vi "Pockels-Mov cor tracing in funct acq.vi"(6 "Cluster":T1={"Pockels ON \"Pre\" (samples)"=2, "Direction (+-Inf)"=enum."No rounding", "Additional duration to stay ON (samples)"=0, "Not the last ROI"=FALSE}, 7 "Actual component time (us)":dbl, 8 "Count towards trigger target (ms) in":dbl, 10 "Excess (us) in":dbl, 11 "Single ROI pockels modulation AO sequence (in)":dbl[](array[numeric])) -> (0 "Count towards trigger target (ms)":dbl, 2 "Excess (us)":dbl, 3 "AO pockels modulation sequence (out)":dbl[](array[numeric]))   [LabVIEW 2020]
uses:
  Typedefs/Pockels modulation Internal cluster 1.ctl
  Typedefs/Rounding type.ctl
  Typedefs/Imaging Protocols enum.ctl
  Globals/gl_Pockels control globals.vi
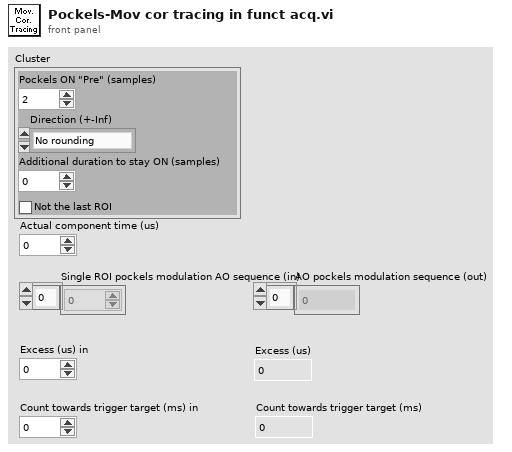
[diagram p1: front panel]
types:
  T1 = typedef "Pockels modulation Internal cluster 1.ctl" = cluster{"Pockels ON \"Pre\" (samples)":i32, "Direction (+-Inf)":T2, "Additional duration to stay ON (samples)":i32, "Not the last ROI":bool}
  T2 = typedef "Rounding type.ctl" = enum16{"No rounding", "Toward +Inf", "Toward -Inf"}
  T3 = typedef "Imaging Protocols enum.ctl" = enum16{"AOL Z-Stack", "Motor Z Stack", "Functional Acquisition", "Single Plane Acquisition", "Volume Acquisition", "Live Imaging", "Live Plane Imaging", "Live Volume Imaging"}
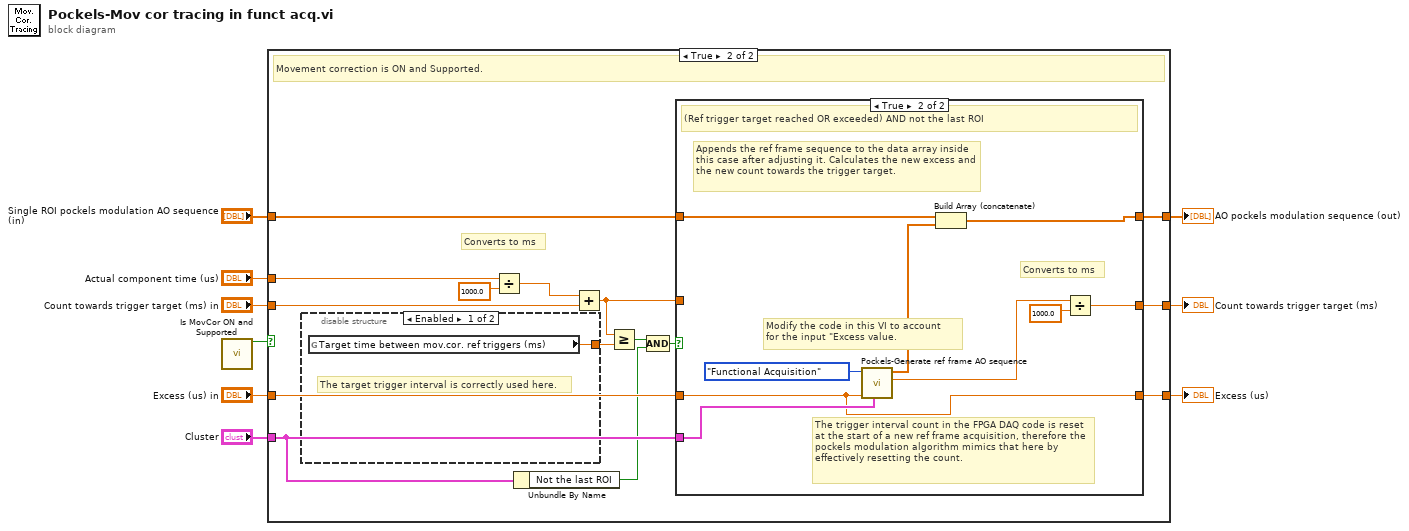
[diagram p0: block diagram]
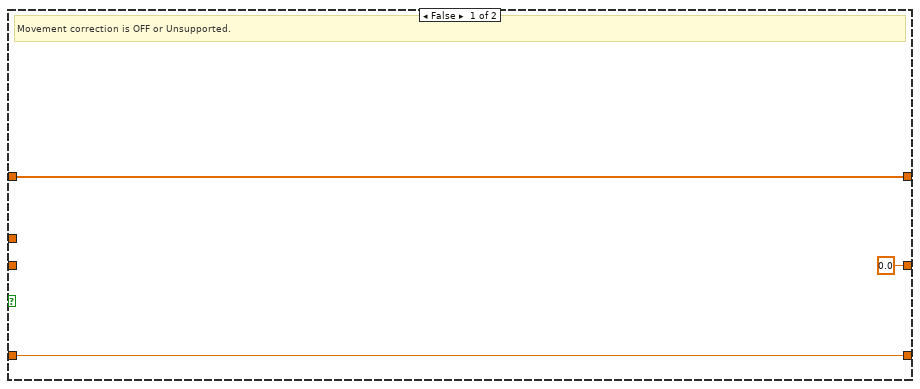
[diagram p2: hidden frame]
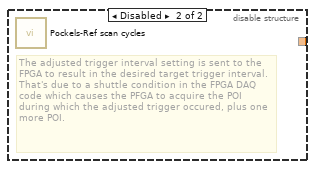
[diagram p3: hidden frame]
diagram:
  n1 = call "Is MovCor ON and Supported.vi"() -> ("MovCor is ON and Supported"=w1:bool)  [unwired: 11 in]
  n2 = case shown="True" w1 {
    tunnel: "Actual component time (us)" -> [_ w26]
    tunnel: "Count towards trigger target (ms) in" -> [_ w24]
    tunnel: "Excess (us) in" -> [w11 w23]
    tunnel: [w11 w22] -> w6
    tunnel: [0.0 w21] -> w5
    tunnel: "Single ROI pockels modulation AO sequence (in)" -> [w12 w20]
    tunnel: [w12 w19] -> w3
    tunnel: "Cluster" -> [_ w14]
    frame False {
      # "Movement correction is OFF or Unsupported."
    }
    frame True {
      # "Converts to ms"
      # "Movement correction is ON and Supported."
      n3 = disable-structure shown="Enabled" {
        disable-tunnel: [w28 _] -> w27
        frame Enabled {
          # "The target trigger interval is correctly used here."
          n4 = global read "gl_Pockels control globals.vi" "Target time between mov.cor. ref triggers (ms)"() -> (w28:dbl)
        }
        frame Disabled {
          # "The adjusted trigger interval setting is sent to the FPGA to result in the desired target trigger interval. That's due to a shuttle condition in the FPGA DAQ code which causes the PFGA to acquire the POI during which the adjusted trigger occured, plus one more POI."
          n5 = call "Pockels-Ref scan cycles.vi"() -> ()  [unwired: 10 in, 2 out]
        }
      }
      n6 = Divide(x=w26, y=1000.0) -> (x/y=w18:dbl)
      n7 = Unbundle By Name(w14) -> ("Not the last ROI"=w13:bool)
      n8 = Add(x=w18, y=w24) -> (x+y=w17:dbl)
      n9 = Greater Or Equal?(x=w17, y=w27) -> (x >= y?=w16:bool)
      n10 = Compound Arithmetic op=AND(w16, w13) -> (w15:bool)
      n11 = case shown="True" w15 {
        tunnel: w23 -> [w31 w32]
        tunnel: [w31 w32] -> w22
        tunnel: w17 -> [w30 _]
        tunnel: [w30 w36] -> w21
        tunnel: w20 -> [w29 w34]
        tunnel: [w29 w39] -> w19
        tunnel: w14 -> [_ w35]
        frame False {
          # "Trigger target not reached"
        }
        frame True {
          # "The trigger interval count in the FPGA DAQ code is reset at the start of a new ref frame acquisition, therefore the pockels modulation algorithm mimics that here by effectively resetting the count."
          # "Converts to ms"
          # "Appends the ref frame sequence to the data array inside this case after adjusting it. Calculates the new excess and the new count towards the trigger target."
          # "Modify the code in this VI to account\nfor the input \"Excess value."
          # "(Ref trigger target reached OR exceeded) AND not the last ROI"
          n12 = call "Pockels-Generate ref frame AO sequence.vi"("Cluster"=w35, "Previous excess us (us)"=w32, "Imaging Protocol"=Imaging_Protocols_enum."Functional Acquisition") -> ("Theoretical acquisition duration of ref frame (us)"=w33:dbl, "Pockels modulation sequence"=w38:dbl[])  [unwired: 4 in, 3 out]
          n13 = Build Array (concatenate)(w34, w38) -> (w39:dbl[])
          n14 = Divide(x=w33, y=1000.0) -> (x/y=w36:dbl)
        }
      }
    }
  }
  "Count towards trigger target (ms)" <- w5
  "Excess (us)" <- w6
  "AO pockels modulation sequence (out)" <- w3
